vi "DAQmx_set_0_AO.vi"(0 "Refnum in":refnum<k21>, 11 "error in (no error)":errorcluster) -> (4 "Refnum out":refnum<k21>, 15 "error out":errorcluster)   [LabVIEW 2017]
uses:
  <vilib>/DAQmx/write.llb/DAQmx Write (Analog DBL 1Chan 1Samp).vi
  <vilib>/DAQmx/configure/timing.llb/DAQmx Timing (Sample Clock).vi
  <vilib>/DAQmx/miscellaneous.llb/DAQmx Fill In Error Info.vi
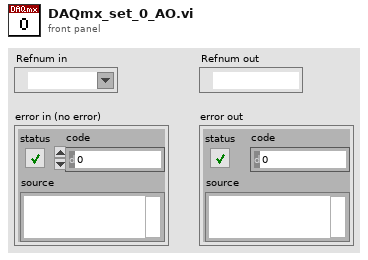
[diagram p1: front panel]
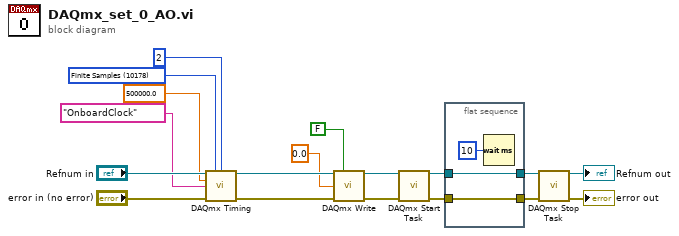
[diagram p0: block diagram]
diagram:
  w7 = 10178 items=["Finite Samples"=10178, "Continuous Samples"=10123, "Hardware Timed Single Point"=12522] ("Sample Mode")
  n1 = call-poly <vilib>:"DAQmx Timing.vi"("task/channels in"="Refnum in", "sample mode"=w7, "samples per channel"=2, "rate"=500000.0, "source"=tag "OnboardClock", "error in"="error in (no error)") -> ("task out"=w13:refnum<k21>, "error out"=w14:errorcluster)  [unwired: 8 in]
  n2 = call-poly <vilib>:"DAQmx Write.vi"("task/channels in"=w13, "auto start"=FALSE, "data"=0.0, "error in"=w14) -> ("task out"=w5:refnum<k21>, "error out"=w6:errorcluster)  [unwired: 9 in, 1 out]
  n3 = call <vilib>:"DAQmx Start Task.vi"("task/channels in"=w5, "error in"=w6) -> ("task out"=w15:refnum<k21>, "error out"=w17:errorcluster)  [unwired: 12 in]
  n4 = flat-sequence {
    tunnel: w15 -> [w21]
    tunnel: [w21] -> w16
    tunnel: w17 -> [w20]
    tunnel: [w20] -> w18
    frame #0 {
      n5 = Wait (ms)(milliseconds to wait=u32 10) -> ()  [unwired: 1 out]
    }
  }
  n6 = call <vilib>:"DAQmx Stop Task.vi"("task/channels in"=w16, "error in"=w18) -> ("task out"=→"Refnum out":refnum<k21>, "error out"=→"error out":errorcluster)  [unwired: 12 in]
